vi "2023 Create Arm Reach Spreadsheet.vi"(0 "error in":errorcluster) -> (1 "transposed array":dbl[][](array[numeric]), 2 "armReachSpreadSheet":string[][](array[string]), 3 "output array 2":dbl[](array[numeric]), 4 "error out":errorcluster)   [LabVIEW 2020]
uses:
  <vilib>/Utility/file.llb/Read Delimited Spreadsheet (string).vi
  2023ArmReachSpreadsheetGlobal.vi
panel:
  out "appended array":dbl[][](array[numeric])
  out "output array":dbl[](array[numeric])
  out "value":dbl
  out "element 2":string
  in  "file path for Win":path=path "C:/git/981LabViewComponents/ArmReachSpreadsheet.csv"
  in  "file path for linux":path=path "/home/lvuser/ArmReachSpreadsheet.csv"
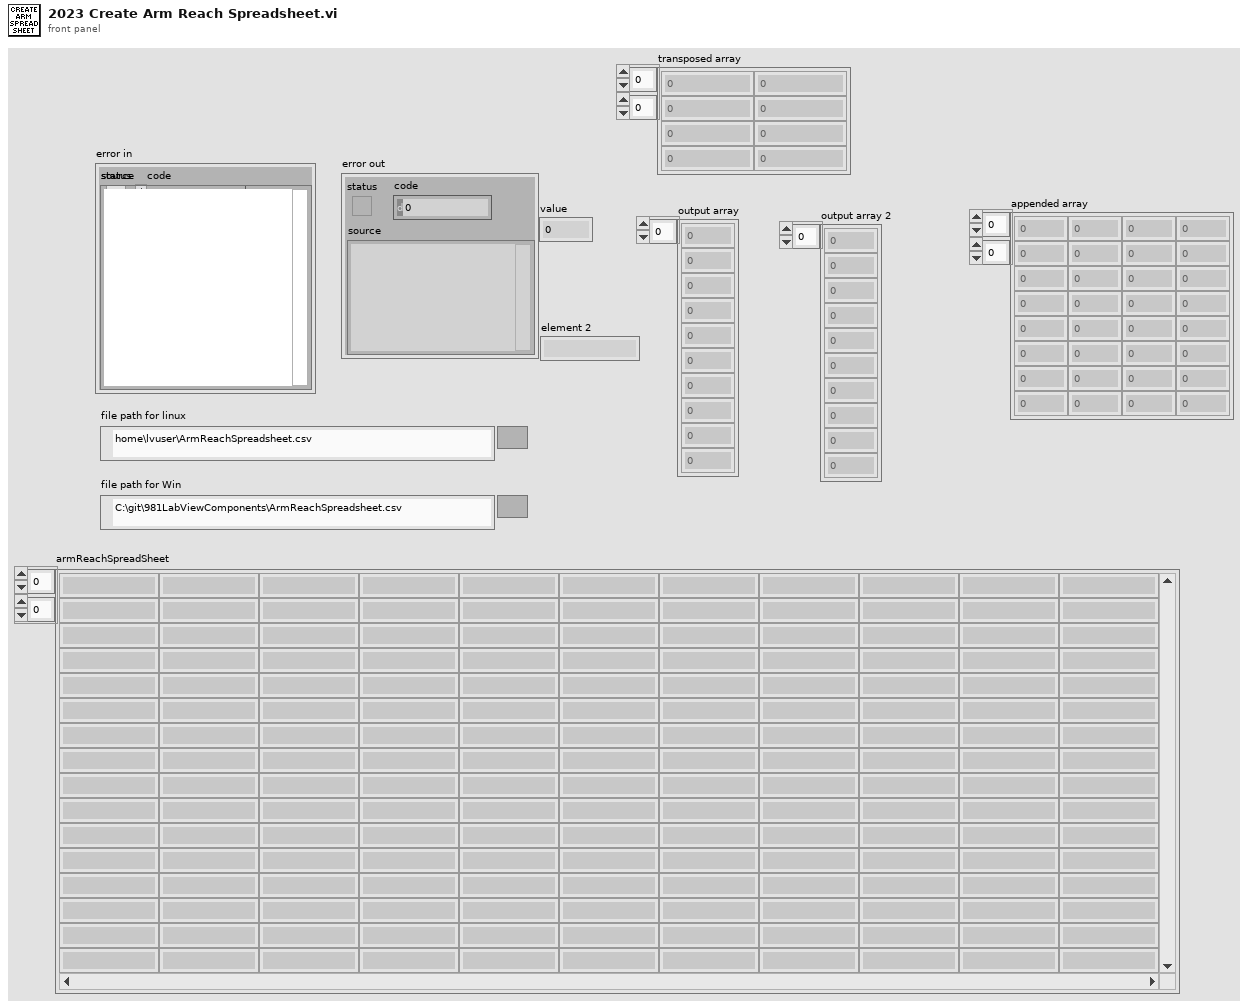
[diagram p1: front panel]
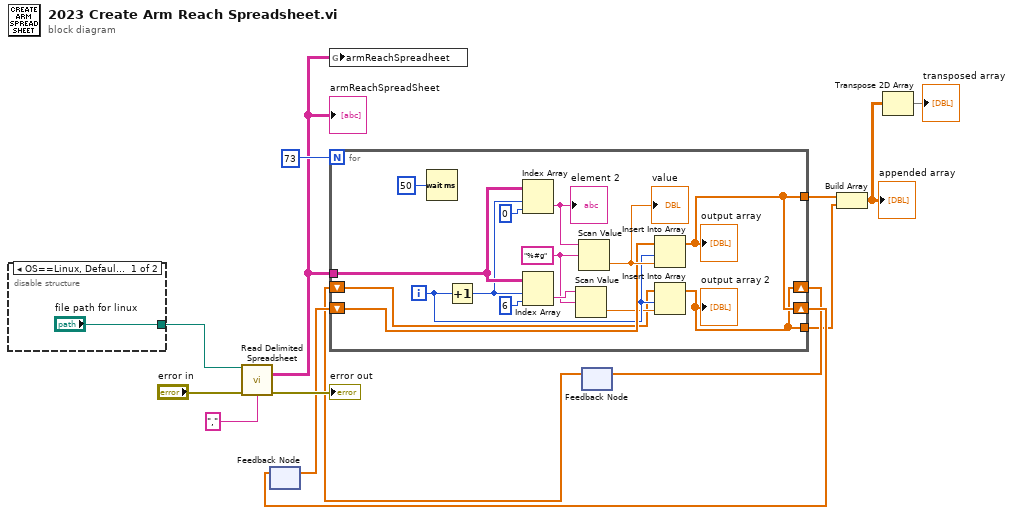
[diagram p0: block diagram]
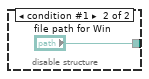
[diagram p2: hidden frame]
diagram:
  n1 = disable-structure shown="OS==Linux, Default" {
    disable-tunnel: ["file path for linux" "file path for Win"] -> w12
    frame condition #0 (active) {
    }
    frame condition #1 {
    }
  }
  n2 = call-poly <vilib>:"Read Delimited Spreadsheet.vi"("file path (dialog if empty)"=w12, "error in (no error)"="error in", "delimiter (\\t)"="," ("delimiter (\\t)")) -> ("all rows"=w1:string[][], "error out"=→"error out":errorcluster)  [unwired: 7 in, 4 out]
  "armReachSpreadSheet" <- w1
  n3 = feedback #1() -> (w8:dbl[])  [unwired: 1 in]
  n4 = global write "2023ArmReachSpreadsheetGlobal.vi" "armReachSpreadheet"(w1) -> ()
  n5 = feedback #2() -> (w6:dbl[])  [unwired: 1 in]
  n6 = for {
    N: 73 -> [_]
    tunnel: w1 -> [w26]
    shift-right: [w18] -> w9
    shift-left: w8 -> [w27]
    shift-right: [w17] -> w7
    shift-left: w6 -> [w19]
    tunnel: [w18] -> w5
    tunnel: [w17] -> w4
    i -> [w21]
    w22 = "%#g" ("format string")
    n7 = Wait (ms)(milliseconds to wait=u32 50) -> ()  [unwired: 1 out]
    n8 = Increment(x=w21) -> (x+1=w25:i32)
    n9 = Index Array(array=w26, index (row)=w25, index (col)=0 ("disabled index (col)")) -> (element=w29:string)
    "element 2" <- w29
    n10 = Index Array(array=w26, index (row)=w25, index (col)=6 ("disabled index (col)")) -> (element=w23:string)
    n11 = Scan Value(string=w23, format string=w22) -> (value=w20:dbl)  [unwired: 1 in, 1 out]
    n12 = Scan Value(string=w29, format string=w22) -> (value=w28:dbl)  [unwired: 1 in, 1 out]
    "value" <- w28
    n13 = Insert Into Array(array=w27, index=w21, new element=w28) -> (w18:dbl[])
    "output array" <- w18
    n14 = Insert Into Array(array=w19, index=w21, new element=w20) -> (w17:dbl[])
    "output array 2" <- w17
  }
  n15 = feedback-in #1(w9) -> ()
  n16 = feedback-in #2(w7) -> ()
  n17 = Build Array(w5, w4) -> (w3:dbl[][])
  "appended array" <- w3
  n18 = Transpose 2D Array(2D array=w3) -> (transposed array=→"transposed array":dbl[][])
